vi "temp test.vi"() -> ()   [LabVIEW 2019]
doc: "This VI captures the region of the screen and displays it on the front panel continuously.\nCan be used to develop remote desktop applications."
uses:
  System.Drawing
  <vilib>/wsapi/NI_WebServices.lvlib
  <vilib>/Utility/miscctls.llb/LVBoundsTypeDef.ctl
  <vilib>/Utility/inputDevices.llb/closeMouse.vi
  <vilib>/Instr/_visa.llb/VISA Configure Serial Port (Instr).vi
  <vilib>/Utility/inputDevices.llb/mouseAcquire.vi
panel:
  out "TX":bool
  out "Scan Cycle":dbl
  out "Disable Timing":bool
  out "VISA":refnum<visa-resource-name>
  out "COM Status":bool
  in  "MC COM Port":refnum<visa-resource-name>="COM5"
  out "MLE Output":string
  out "Possible Inputs":string[](array[string])
  out "Input Likelihood":dbl[](array[numeric])
  out "Max Index":i32
  out "Write String":string
  in  "Timing Detected":bool
  out "Disable Space":bool
  out "Match Score":i32
  in  "Match Threshold":dbl=800.0
  out "Valid Range":bool
  in  "Error In 3":errorcluster
  in  "Space Detected":bool
  in  "Error In 2":errorcluster
  out "Post Processed Combo":picture
  in  "delay":u32=100
  in  "Error In":errorcluster
  out "Raw OCR Output":string
  in  "Combo y offset":i32=150
  in  "Combo x offset":i32=-100
  out "Combo":picture
  in  "Combo  Height  (px)":i32=50
  in  "Combo Width (px)":i32=360
  in  "Bar y offset":i32=200
  in  "Bar x offset":i32=-70
  out "Bar":picture
  in  "Bar Height  (px)":i32=30
  in  "Bar Width (px)":i32=280
  in  "Space Height (px)":i32=60
  in  "Space Width (px)":i32=145
  out "Space":picture
  in  "stop":bool
  # "Controls, Parameters, and Debug"
  # "Space Initiation"
  # "Bar Timing"
  # "Combo OCR"
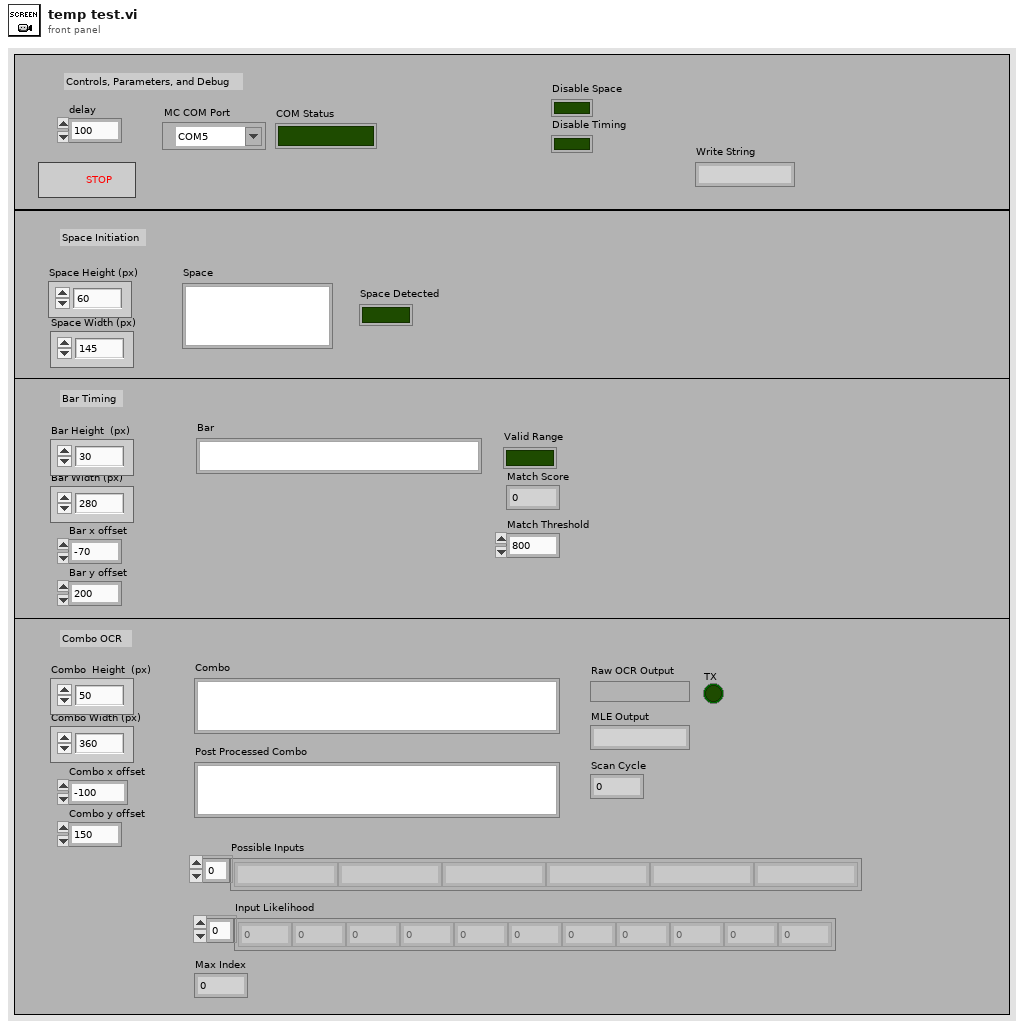
[diagram p1: front panel]
types:
  T1 = typedef "LVBoundsTypeDef.ctl" = cluster{"Width":u32, "Height":u32}
  T2 = typedef "Image Type" = u32
  T3 = cluster{"Horizontal":i32, "Vertical":i32, "Scrolling":i32}
  T4 = typedef "IMAQ Image.ctl" = refnum<image>
  T5 = typedef "imagedata.ctl" = cluster{"image type":i32, "image depth":i32, "image":u8[], "mask":u8[], "colors":u32[], "Rectangle":cluster{"left":i16, "top":i16, "right":i16, "bottom":i16}}
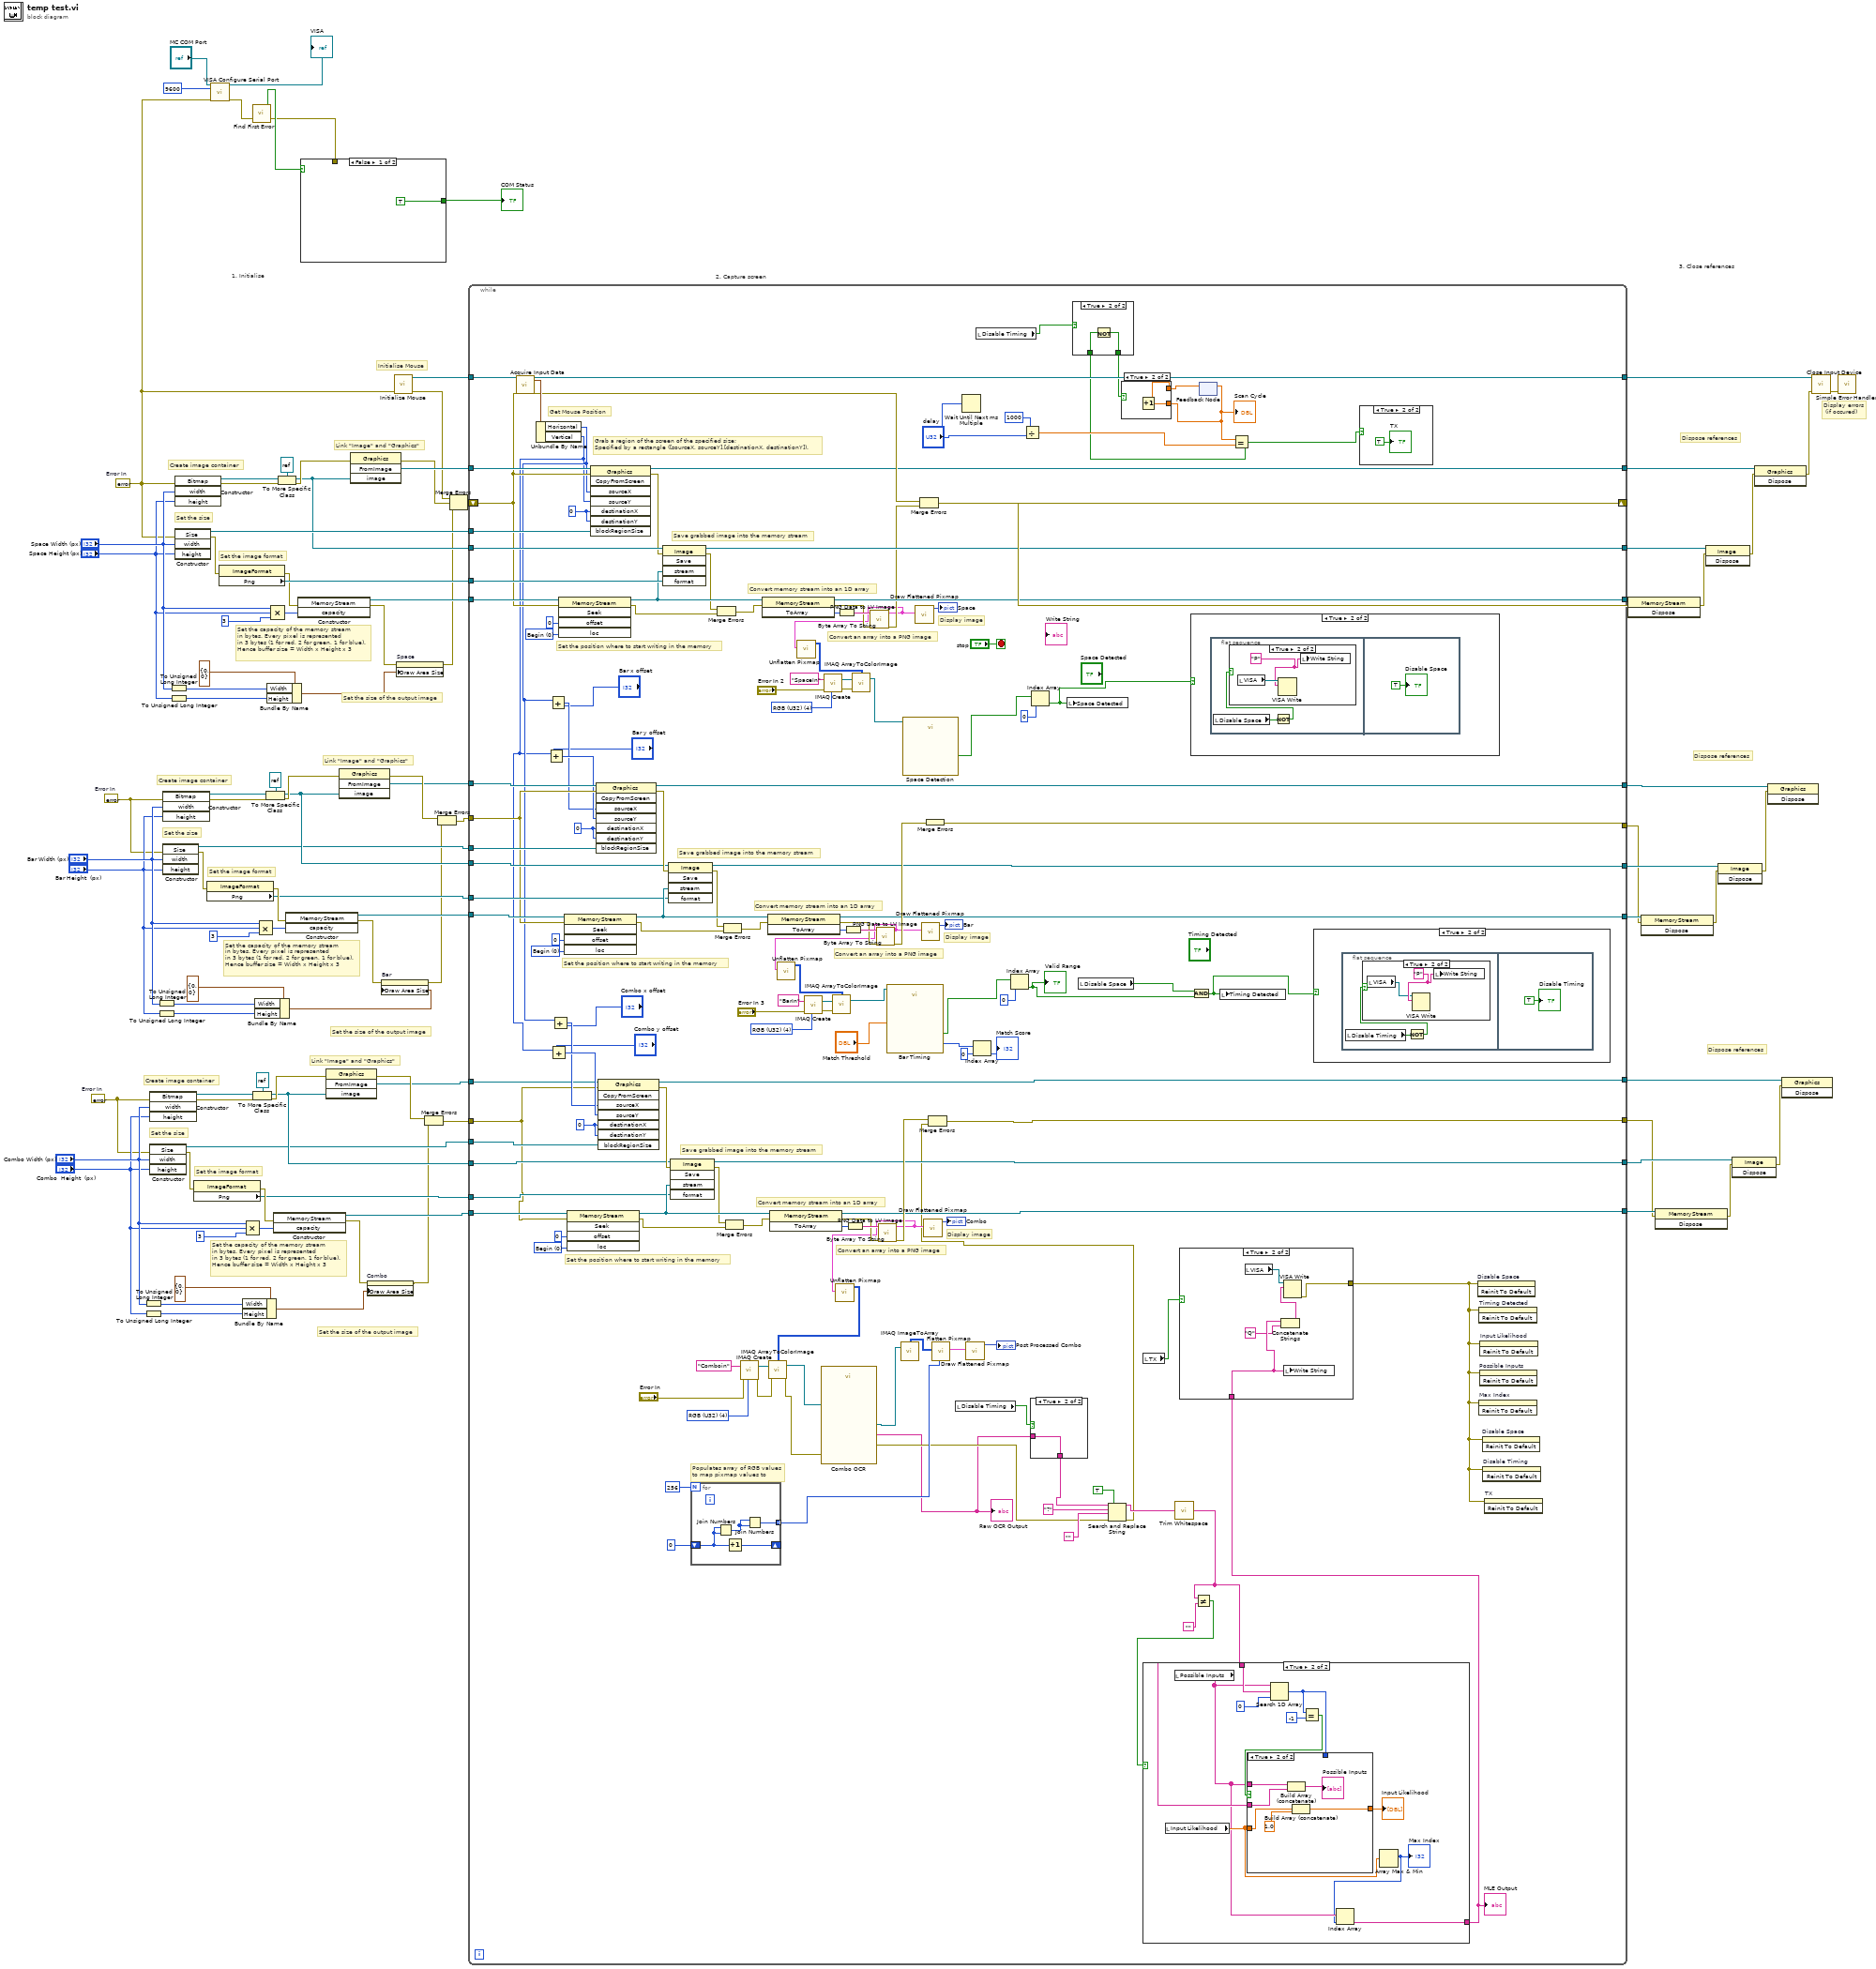
[diagram p0: block diagram]
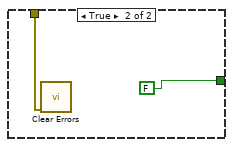
[diagram p2: hidden frame]
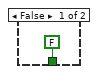
[diagram p4: hidden frame]
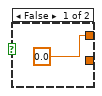
[diagram p5: hidden frame]
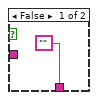
[diagram p11: hidden frame]
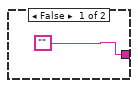
[diagram p12: hidden frame]
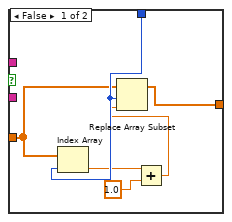
[diagram p13: hidden frame]
diagram:
  w24 = errorcluster {"status"=FALSE, "code"=0, "source"=""}  # Error In
  w54 = errorcluster {"status"=FALSE, "code"=0, "source"=""}  # Error In
  w2 = errorcluster {"status"=FALSE, "code"=0, "source"=""}  # Error In
  # "Dispose references"
  # "Link \"Image\" and \"Graphics\""
  # "Set the size"
  # "Create image container"
  # "Set the image format"
  # "Set the size of the output image"
  # "Set the capacity of the memory stream\nin bytes. Every pixel is represented\nin 3 bytes (1 for red, 2 for green, 1 for blue).\nHence buffer size = Width x Height x 3"
  # "Dispose references"
  # "Link \"Image\" and \"Graphics\""
  # "Set the size"
  # "Create image container"
  # "Set the image format"
  # "Set the size of the output image"
  # "Set the capacity of the memory stream\nin bytes. Every pixel is represented\nin 3 bytes (1 for red, 2 for green, 1 for blue).\nHence buffer size = Width x Height x 3"
  # "Link \"Image\" and \"Graphics\""
  # "Set the size"
  # "Create image container"
  # "3. Close references"
  # "2. Capture screen"
  # "1. Initialise"
  # "Display errors\n (if occured)"
  # "Dispose references"
  # "Set the image format"
  # "Set the size of the output image"
  # "Set the capacity of the memory stream\nin bytes. Every pixel is represented\nin 3 bytes (1 for red, 2 for green, 1 for blue).\nHence buffer size = Width x Height x 3"
  # "Initialise Mouse"
  n1 = To Unsigned Long Integer(number="Combo Width (px)") -> (unsigned 32bit integer=w27:u32)
  n2 = To Unsigned Long Integer(number="Combo  Height  (px)") -> (unsigned 32bit integer=w25:u32)
  n3 = constructor class="Bitmap"(error in=w24, "width"="Combo Width (px)", "height"="Combo  Height  (px)") -> (reference out=w35:refnum<k24>, error out=w37:errorcluster)  [unwired: 2 in, 3 out]
  n4 = constructor class="Size"(error in=w24, "width"="Combo Width (px)", "height"="Combo  Height  (px)") -> (reference out=w20:refnum<k24>, error out=w31:errorcluster)  [unwired: 2 in, 3 out]
  n5 = To Unsigned Long Integer(number="Bar Width (px)") -> (unsigned 32bit integer=w57:u32)
  n6 = To Unsigned Long Integer(number="Bar Height  (px)") -> (unsigned 32bit integer=w55:u32)
  n7 = constructor class="Bitmap"(error in=w54, "width"="Bar Width (px)", "height"="Bar Height  (px)") -> (reference out=w65:refnum<k24>, error out=w67:errorcluster)  [unwired: 2 in, 3 out]
  n8 = constructor class="Size"(error in=w54, "width"="Bar Width (px)", "height"="Bar Height  (px)") -> (reference out=w50:refnum<k24>, error out=w61:errorcluster)  [unwired: 2 in, 3 out]
  n9 = To Unsigned Long Integer(number="Space Width (px)") -> (unsigned 32bit integer=w76:u32)
  n10 = To Unsigned Long Integer(number="Space Height (px)") -> (unsigned 32bit integer=w74:u32)
  n11 = constructor class="Bitmap"(error in=w2, "width"="Space Width (px)", "height"="Space Height (px)") -> (reference out=w96:refnum<k24>, error out=w99:errorcluster)  [unwired: 2 in, 3 out]
  n12 = constructor class="Size"(error in=w2, "width"="Space Width (px)", "height"="Space Height (px)") -> (reference out=w94:refnum<k24>, error out=w85:errorcluster)  [unwired: 2 in, 3 out]
  n13 = property class="ImageFormat"(error in=w31) -> (error out=w30:errorcluster, "Png"=w22:refnum<k24>)  [unwired: 1 in, 1 out]
  n14 = property class="ImageFormat"(error in=w61) -> (error out=w60:errorcluster, "Png"=w52:refnum<k24>)  [unwired: 1 in, 1 out]
  n15 = call-poly "VISA Configure Serial Port"("VISA resource name"="MC COM Port", "baud rate (9600)"=u32 9600, "error in (no error)"=w2) -> ("VISA resource name out"=→"VISA":refnum<visa-resource-name>, "error out"=w7:errorcluster)  [unwired: 11 in]
  n16 = property class="ImageFormat"(error in=w85) -> (error out=w84:errorcluster, "Png"=w93:refnum<k24>)  [unwired: 1 in, 1 out]
  n17 = Bundle By Name(cluster=T1 {"Width"=0, "Height"=0} ("Draw Area Size"), "Width"=w27, "Height"=w25) -> (w11:T1)
  n18 = Compound Arithmetic op=MULTIPLY("Combo Width (px)", "Combo  Height  (px)", 3 ("value")) -> (w33:i32)
  n19 = call <vilib>:"Find First Error.vi"("error in (no error)"=w7) -> ("error out"=w4:errorcluster, "error?"=w6:bool)  [unwired: 3 in]
  n20 = To More Specific Class(target class=refnum<k24> refnum, reference=w35, error in=w37) -> (specific class reference=w21:refnum<k24>, error out=w38:errorcluster)
  n21 = Bundle By Name(cluster=T1 {"Width"=0, "Height"=0} ("Draw Area Size"), "Width"=w57, "Height"=w55) -> (w39:T1)
  n22 = Compound Arithmetic op=MULTIPLY("Bar Width (px)", "Bar Height  (px)", 3 ("value")) -> (w63:i32)
  n23 = To More Specific Class(target class=refnum<k24> refnum, reference=w65, error in=w67) -> (specific class reference=w51:refnum<k24>, error out=w68:errorcluster)
  n24 = Bundle By Name(cluster=T1 {"Width"=0, "Height"=0} ("Draw Area Size"), "Width"=w76, "Height"=w74) -> (w80:T1)
  n25 = Compound Arithmetic op=MULTIPLY("Space Width (px)", "Space Height (px)", 3 ("value")) -> (w88:i32)
  n26 = constructor class="MemoryStream"(error in=w30, "capacity"=w33) -> (reference out=w23:refnum<k24>, error out=w10:errorcluster)  [unwired: 2 in, 2 out]
  n27 = To More Specific Class(target class=refnum<k24> refnum, reference=w96, error in=w99) -> (specific class reference=w87:refnum<k24>, error out=w100:errorcluster)
  n28 = constructor class="MemoryStream"(error in=w60, "capacity"=w63) -> (reference out=w53:refnum<k24>, error out=w40:errorcluster)  [unwired: 2 in, 2 out]
  n29 = constructor class="MemoryStream"(error in=w84, "capacity"=w88) -> (reference out=w90:refnum<k24>, error out=w79:errorcluster)  [unwired: 2 in, 2 out]
  n30 = case shown="False" w6 {
    tunnel: [TRUE FALSE] -> w5
    tunnel: w4 -> [_ w104]
    frame False {
    }
    frame True {
      n31 = call <vilib>:"Clear Errors.vi"("error in (no error)"=w104) -> ()  [unwired: 5 in, 2 out]
    }
  }
  "COM Status" <- w5
  n32 = invoke class="Graphics" method="FromImage"(error in=w38, "image"=w21) -> (error out=w29:errorcluster, "FromImage"=w19:refnum<k24>)  [unwired: 2 in, 2 out]
  n33 = invoke class="Graphics" method="FromImage"(error in=w68, "image"=w51) -> (error out=w59:errorcluster, "FromImage"=w49:refnum<k24>)  [unwired: 2 in, 2 out]
  n34 = invoke class="Graphics" method="FromImage"(error in=w100, "image"=w87) -> (error out=w83:errorcluster, "FromImage"=w97:refnum<k24>)  [unwired: 2 in, 2 out]
  n35 = property on="Combo" class="Pict"(error in=w10, "Draw Area Size"=w11) -> (error out=w9:errorcluster)  [unwired: 1 in, 1 out]
  n36 = property on="Bar" class="Pict"(error in=w40, "Draw Area Size"=w39) -> (error out=w41:errorcluster)  [unwired: 1 in, 1 out]
  n37 = call <vilib>:"Initialize Mouse.vi"("error in (no error)"=w2) -> ("error out"=w81:errorcluster, "device ID"=w102:refnum<k1>)  [unwired: 9 in]
  n38 = property on="Space" class="Pict"(error in=w79, "Draw Area Size"=w80) -> (error out=w78:errorcluster)  [unwired: 1 in, 1 out]
  n39 = Merge Errors(w29, w9) -> (w18:errorcluster)
  n40 = Merge Errors(w59, w41) -> (w48:errorcluster)
  n41 = Merge Errors(w81, w83, w78) -> (w82:errorcluster)
  n42 = while {
    tunnel: w102 -> [w256]
    tunnel: [w254] -> w101
    tunnel: w97 -> [w253]
    tunnel: [w250] -> w95
    tunnel: w94 -> [w249]
    tunnel: w93 -> [w248]
    tunnel: [w247] -> w92
    tunnel: w90 -> [w246]
    tunnel: w87 -> [w239]
    shift-right: [w230] -> w73
    shift-left: w82 -> [w233]
    tunnel: [w229] -> w72
    tunnel: w53 -> [w215]
    tunnel: w52 -> [w214]
    tunnel: w51 -> [w213]
    tunnel: w50 -> [w212]
    tunnel: w49 -> [w211]
    tunnel: w48 -> [w210]
    tunnel: [w209] -> w45
    tunnel: [w208] -> w44
    tunnel: [w207] -> w43
    tunnel: [w206] -> w42
    tunnel: w23 -> [w184]
    tunnel: w22 -> [w183]
    tunnel: w21 -> [w182]
    tunnel: w20 -> [w181]
    tunnel: w19 -> [w180]
    tunnel: w18 -> [w179]
    tunnel: [w176] -> w15
    tunnel: [w175] -> w14
    tunnel: [w174] -> w13
    tunnel: [w173] -> w12
    stop <- "stop" stop-if-true
    w146 = T2 4 items=["Grayscale (U8)", "Grayscale (I16)", "Grayscale (SGL)", "Complex (CSG)", "RGB (U32)", "HSL (U32)", "RGB (U64)", "Grayscale (U16)"] ("Image Type")
    w157 = T2 4 items=["Grayscale (U8)", "Grayscale (I16)", "Grayscale (SGL)", "Complex (CSG)", "RGB (U32)", "HSL (U32)", "RGB (U64)", "Grayscale (U16)"] ("Image Type")
    w172 = T2 4 items=["Grayscale (U8)", "Grayscale (I16)", "Grayscale (SGL)", "Complex (CSG)", "RGB (U32)", "HSL (U32)", "RGB (U64)", "Grayscale (U16)"] ("Image Type")
    w195 = 0 ("destinationX")
    w198 = 0 items=["Begin", "Current", "End"] ("loc")
    w222 = 0 ("destinationX")
    w225 = 0 items=["Begin", "Current", "End"] ("loc")
    w240 = 0 ("destinationX")
    w244 = 0 items=["Begin", "Current", "End"] ("loc")
    # "Populates array of RGB values\nto map pixmap values to"
    # "Display image"
    # "Convert an array into a PNG image"
    # "Set the position where to start writing in the memory"
    # "Convert memory stream into an 1D array"
    # "Save grabbed image into the memory stream"
    # "Display image"
    # "Convert an array into a PNG image"
    # "Set the position where to start writing in the memory"
    # "Convert memory stream into an 1D array"
    # "Save grabbed image into the memory stream"
    # "Display image"
    # "Convert an array into a PNG image"
    # "Set the position where to start writing in the memory"
    # "Convert memory stream into an 1D array"
    # "Save grabbed image into the memory stream"
    # "Grab a region of the screen of the specified size;\nSpecified by a rectangle ([sourceX, sourceY],[destinationX, destinationY])."
    # "Get Mouse Position"
    n43 = call-poly <vilib>:"Acquire Input Data.vi"("device ID"=w256, "error in (no error)"=w233) -> ("device ID"=w254:refnum<k1>, "axis info"=w255:T3, "error out"=w232:errorcluster)  [unwired: 14 in, 1 out]
    n44 = Unbundle By Name(w255) -> ("Horizontal"=w178:i32, "Vertical"=w177:i32)
    n45 = Add(x=w177, y="Bar y offset") -> (x+y=w205:i32)
    n46 = Add(x=w178, y="Bar x offset") -> (x+y=w204:i32)
    n47 = Add(x=w177, y="Combo y offset") -> (x+y=w188:i32)
    n48 = Add(x=w178, y="Combo x offset") -> (x+y=w187:i32)
    n49 = invoke class="MemoryStream" method="Seek"(reference=w246, error in=w233, "offset"=i64 0, "loc"=w244) -> (reference out=w241:refnum<k24>, error out=w236:errorcluster)  [unwired: 1 in, 3 out]
    n50 = invoke class="MemoryStream" method="Seek"(reference=w215, error in=w210, "offset"=i64 0, "loc"=w225) -> (reference out=w223:refnum<k24>, error out=w219:errorcluster)  [unwired: 1 in, 3 out]
    n51 = invoke class="MemoryStream" method="Seek"(reference=w184, error in=w179, "offset"=i64 0, "loc"=w198) -> (reference out=w196:refnum<k24>, error out=w192:errorcluster)  [unwired: 1 in, 3 out]
    n52 = invoke class="Graphics" method="CopyFromScreen"(reference=w253, error in=w233, "sourceX"=w178, "sourceY"=w177, "destinationX"=w240, "destinationY"=w240, "blockRegionSize"=w249) -> (reference out=w229:refnum<k24>, error out=w234:errorcluster)  [unwired: 1 in, 6 out]
    n53 = invoke class="Graphics" method="CopyFromScreen"(reference=w211, error in=w210, "sourceX"=w204, "sourceY"=w205, "destinationX"=w222, "destinationY"=w222, "blockRegionSize"=w212) -> (reference out=w208:refnum<k24>, error out=w217:errorcluster)  [unwired: 1 in, 6 out]
    n54 = invoke class="Graphics" method="CopyFromScreen"(reference=w180, error in=w179, "sourceX"=w187, "sourceY"=w188, "destinationX"=w195, "destinationY"=w195, "blockRegionSize"=w181) -> (reference out=w173:refnum<k24>, error out=w190:errorcluster)  [unwired: 1 in, 6 out]
    n55 = invoke class="Image" method="Save"(reference=w239, error in=w234, "stream"=w241, "format"=w248) -> (reference out=w247:refnum<k24>, error out=w237:errorcluster)  [unwired: 1 in, 3 out]
    n56 = invoke class="Image" method="Save"(reference=w213, error in=w217, "stream"=w223, "format"=w214) -> (reference out=w209:refnum<k24>, error out=w220:errorcluster)  [unwired: 1 in, 3 out]
    n57 = invoke class="Image" method="Save"(reference=w182, error in=w190, "stream"=w196, "format"=w183) -> (reference out=w175:refnum<k24>, error out=w193:errorcluster)  [unwired: 1 in, 3 out]
    n58 = for {
      N: 256 -> [_]
      tunnel: [w307] -> w158 mode=indexing
      shift-right: [w306] -> _
      shift-left: u8 0 -> [w304]
      n59 = Join Numbers(hi=w304, lo=w304) -> ((hi.lo)=w305:u16)
      n60 = Increment(x=w304) -> (x+1=w306:u8)
      n61 = Join Numbers(hi=w305, lo=w305) -> ((hi.lo)=w307:u32)
    }
    n62 = Merge Errors(w237, w236) -> (w235:errorcluster)
    n63 = Merge Errors(w220, w219) -> (w218:errorcluster)
    n64 = Merge Errors(w193, w192) -> (w191:errorcluster)
    n65 = call "IMAQ Create"("Image Name"="Comboin", "Image Type"=w172, "error in (no error)"="Error In") -> ("New Image"=w171:T4, "error out"=w170:errorcluster)  [unwired: 1 in, 1 out]
    n66 = invoke class="MemoryStream" method="ToArray"(reference=w241, error in=w235) -> (reference out=w250:refnum<k24>, error out=w238:errorcluster, "ToArray"=w252:u8[])  [unwired: 1 in]
    n67 = invoke class="MemoryStream" method="ToArray"(reference=w223, error in=w218) -> (reference out=w207:refnum<k24>, error out=w221:errorcluster, "ToArray"=w228:u8[])  [unwired: 1 in]
    n68 = invoke class="MemoryStream" method="ToArray"(reference=w196, error in=w191) -> (reference out=w176:refnum<k24>, error out=w194:errorcluster, "ToArray"=w201:u8[])  [unwired: 1 in]
    n69 = call "IMAQ Create"("Image Name"="BarIn", "Image Type"=w146, "error in (no error)"="Error In 3") -> ("New Image"=w145:T4, "error out"=w144:errorcluster)  [unwired: 1 in, 1 out]
    n70 = call "IMAQ Create"("Image Name"="SpaceIn", "Image Type"=w157, "error in (no error)"="Error In 2") -> ("New Image"=w156:T4, "error out"=w155:errorcluster)  [unwired: 1 in, 1 out]
    n71 = Byte Array To String(unsigned byte array=w252) -> (string=w251:string)
    n72 = Byte Array To String(unsigned byte array=w228) -> (string=w227:string)
    n73 = Byte Array To String(unsigned byte array=w201) -> (string=w200:string)
    n74 = call <vilib>:"PNG Data to LV Image.vi"("error in (no error)"=w238, "png data"=w251) -> ("error out"=w231:errorcluster, "image data"=w153:T5)  [unwired: 8 in]
    n75 = call <vilib>:"Unflatten Pixmap.vi"("image data"=w153) -> ("24-bit pixmap"=w152:u32[][])  [unwired: 4 in, 6 out]
    n76 = call "IMAQ ArrayToColorImage"("Image Pixels (U32)"=w152, "Image"=w156, "error in (no error)"=w155) -> ("Image Out"=w151:T4)  [unwired: 2 in, 1 out]
    n77 = call <vilib>:"PNG Data to LV Image.vi"("error in (no error)"=w221, "png data"=w227) -> ("error out"=w216:errorcluster, "image data"=w140:T5)  [unwired: 8 in]
    n78 = call <vilib>:"Unflatten Pixmap.vi"("image data"=w140) -> ("24-bit pixmap"=w139:u32[][])  [unwired: 4 in, 6 out]
    n79 = call "IMAQ ArrayToColorImage"("Image Pixels (U32)"=w139, "Image"=w145, "error in (no error)"=w144) -> ("Image Out"=w141:T4)  [unwired: 2 in, 1 out]
    n80 = call <vilib>:"PNG Data to LV Image.vi"("error in (no error)"=w194, "png data"=w200) -> ("error out"=w189:errorcluster, "image data"=w167:T5)  [unwired: 8 in]
    n81 = call <vilib>:"Unflatten Pixmap.vi"("image data"=w167) -> ("24-bit pixmap"=w166:u32[][])  [unwired: 4 in, 6 out]
    n82 = call "IMAQ ArrayToColorImage"("Image Pixels (U32)"=w166, "Image"=w171, "error in (no error)"=w170) -> ("Image Out"=w168:T4, "error out"=w169:errorcluster)  [unwired: 2 in]
    n83 = call "Combo OCR"("Image In"=w168, "error in"=w169) -> ("Image Out"=w164:T4, "String (OCR/OCV 2)"=w120:string, "error out"=w128:errorcluster)  [unwired: 23 in]
    "Raw OCR Output" <- w120
    n84 = call "Bar Timing"("Image In"=w141, "Minimum Match Score (Color Matching 1)"="Match Threshold") -> ("Match Flag (Color Matching 1)"=w137:bool[], "Match Score (Color Matching 1)"=w135:i32[])  [unwired: 22 in, 2 out]
    n85 = call "IMAQ ImageToArray"("Image"=w164) -> ("Image Pixels (U8)"=w161:u8[][])  [unwired: 3 in, 4 out]
    n86 = call "Space Detection"("Image In"=w151) -> ("Match Flag (Color Matching 1)"=w148:bool[])  [unwired: 23 in, 3 out]
    n87 = call <vilib>:"Draw Flattened Pixmap.vi"("image data"=w153) -> ("new picture"=→"Space":picture)  [unwired: 8 in]
    n88 = Merge Errors(w232, w231) -> (w230:errorcluster)
    n89 = call <vilib>:"Draw Flattened Pixmap.vi"("image data"=w140) -> ("new picture"=→"Bar":picture)  [unwired: 8 in]
    n90 = call <vilib>:"Draw Flattened Pixmap.vi"("image data"=w167) -> ("new picture"=→"Combo":picture)  [unwired: 8 in]
    n91 = Merge Errors(w216) -> (w206:errorcluster)
    n92 = call <vilib>:"Flatten Pixmap.vi"("colors"=w158, "8-bit pixmap"=w161) -> ("image data"=w162:T5)  [unwired: 9 in]
    n93 = local read "Disable Timing"() -> (w109:bool)
    n94 = Wait Until Next ms Multiple(millisecond multiple="delay") -> ()  [unwired: 1 out]
    n95 = call <vilib>:"Draw Flattened Pixmap.vi"("image data"=w162) -> ("new picture"=→"Post Processed Combo":picture)  [unwired: 8 in]
    n96 = Index Array(array=w135, index=0) -> (element=→"Match Score":i32)
    n97 = local read "Disable Timing"() -> (w110:bool)
    n98 = Index Array(array=w137, index=0) -> (element=w123:bool)
    "Valid Range" <- w123
    n99 = Divide(x=1000, y="delay") -> (x/y=w116:dbl)
    n100 = case shown="True" w109 {
      tunnel: ["" w280] -> w121
      tunnel: w120 -> [_ w280]
      frame False {
      }
      frame True {
      }
    }
    n101 = Index Array(array=w148, index=0) -> (element=w117:bool)
    n102 = local write "Space Detected"(w117) -> ()
    n103 = local read "Disable Space"() -> (w122:bool)
    n104 = Search and Replace String(replace all?=TRUE ("replace all? (F)"), input string=w121, search string="?", replace string="", error in=w128) -> (result string=w129:string, error out=w127:errorcluster)  [unwired: 3 in, 2 out]
    n105 = Merge Errors(w189, w127) -> (w174:errorcluster)
    n106 = local read "TX"() -> (w107:bool)
    n107 = call <vilib>:"Trim Whitespace.vi"("string"=w129) -> ("trimmed string"=w125:string)  [unwired: 1 in]
    n108 = case shown="True" w117 {
      frame False {
      }
      frame True {
        n109 = flat-sequence {
          frame #0 {
            n110 = local read "Disable Space"() -> (w265:bool)
            n111 = Not(x=w265) -> (.not. x?=w264:bool)
            n112 = case shown="True" w264 {
              frame False {
              }
              frame True {
                w266 = "P" ("Write String")
                n113 = local read "VISA"() -> (w267:refnum<visa-resource-name>)
                n114 = VISA Write(VISA resource name=w267, write buffer=w266) -> ()  [unwired: 1 in, 3 out]
                n115 = local write "Write String"(w266) -> ()
              }
            }
          }
          frame #1 {
            "Disable Space" <- TRUE ("Enable Space")
          }
        }
      }
    }
    n116 = And(x=w122, y=w123) -> (x .and. y?=w118:bool)
    n117 = Not Equal?(x=w125, y="") -> (x != y?=w124:bool)
    n118 = case shown="True" w124 {
      tunnel: w125 -> [_ w286]
      tunnel: ["" w282] -> w119
      frame False {
      }
      frame True {
        n119 = local read "Input Likelihood"() -> (w285:dbl[])
        n120 = local read "Possible Inputs"() -> (w284:string[])
        n121 = Search 1D Array(1D array=w284, element=w286, start index (0)=0) -> (index of element=w288:i32)
        n122 = Equal?(x=w288, y=-1) -> (x = y?=w289:bool)
        n123 = case shown="True" w289 {
          tunnel: w284 -> [_ w303]
          tunnel: w286 -> [_ w302]
          tunnel: w288 -> [w297 _]
          tunnel: w285 -> [w293 w299]
          tunnel: [w292 w300] -> w287
          frame False {
            n124 = Index Array(array=w293, index=w297) -> (element=w295:dbl)
            n125 = Add(x=w295, y=1.0) -> (x+y=w294:dbl)
            n126 = Replace Array Subset(array=w293, new element=w294, index=w297) -> (w292:dbl[])
          }
          frame True {
            n127 = Build Array (concatenate)(w303, w302) -> (→"Possible Inputs":string[])
            n128 = Build Array (concatenate)(w299, 1.0 ("new element/subarray")) -> (w300:dbl[])
          }
        }
        "Input Likelihood" <- w287
        n129 = Array Max & Min(array=w285) -> (max index (indices)=w283:i32)  [unwired: 3 out]
        "Max Index" <- w283
        n130 = Index Array(array=w284, index=w283) -> (element=w282:string)
      }
    }
    "MLE Output" <- w119
    n131 = case shown="True" w107 {
      tunnel: w119 -> [_ w273]
      tunnel: [_ w269] -> w106
      frame False {
      }
      frame True {
        n132 = local read "VISA"() -> (w272:refnum<visa-resource-name>)
        n133 = Concatenate Strings(w273, "Q" ("string")) -> (w270:string)
        n134 = VISA Write(VISA resource name=w272, write buffer=w270) -> (error out=w269:errorcluster)  [unwired: 1 in, 2 out]
        n135 = local write "Write String"(w273) -> ()
      }
    }
    n136 = feedback #1() -> (w115:dbl)  [unwired: 1 in]
    "Scan Cycle" <- w115
    n137 = local write "Timing Detected"(w118) -> ()
    n138 = Equal?(x=w115, y=w116) -> (x = y?=w108:bool)
    n139 = case shown="True" w110 {
      tunnel: [FALSE w260] -> w114
      tunnel: w108 -> [_ w259]
      frame False {
      }
      frame True {
        n140 = Not(x=w259) -> (.not. x?=w260:bool)
      }
    }
    n141 = case shown="True" w114 {
      tunnel: [0.0 w263] -> w112
      tunnel: w115 -> [_ w262]
      frame False {
      }
      frame True {
        n142 = Increment(x=w262) -> (x+1=w263:dbl)
      }
    }
    n143 = feedback-in #1(w112) -> ()
    n144 = case shown="True" w118 {
      frame False {
      }
      frame True {
        n145 = flat-sequence {
          frame #0 {
            n146 = local read "Disable Timing"() -> (w275:bool)
            n147 = Not(x=w275) -> (.not. x?=w274:bool)
            n148 = case shown="True" w274 {
              frame False {
              }
              frame True {
                w277 = "P" ("Write String")
                n149 = local read "VISA"() -> (w276:refnum<visa-resource-name>)
                n150 = VISA Write(VISA resource name=w276, write buffer=w277) -> ()  [unwired: 1 in, 3 out]
                n151 = local write "Write String"(w277) -> ()
              }
            }
          }
          frame #1 {
            "Disable Timing" <- TRUE ("Enable Space")
          }
        }
      }
    }
    n152 = case shown="True" w108 {
      frame False {
      }
      frame True {
        "TX" <- TRUE ("TX")
      }
    }
    n153 = invoke on="Disable Space" class="Bool (strict)" method="Reinit To Default"(error in=w106) -> ()  [unwired: 2 in, 3 out]
    n154 = invoke on="Timing Detected" class="Bool (strict)" method="Reinit To Default"(error in=w106) -> ()  [unwired: 2 in, 3 out]
    n155 = invoke on="Max Index" class="DigNum (strict)" method="Reinit To Default"(error in=w106) -> ()  [unwired: 2 in, 3 out]
    n156 = invoke on="Possible Inputs" class="Arr (strict)" method="Reinit To Default"(error in=w106) -> ()  [unwired: 2 in, 3 out]
    n157 = invoke on="Input Likelihood" class="Arr (strict)" method="Reinit To Default"(error in=w106) -> ()  [unwired: 2 in, 3 out]
    n158 = invoke on="Disable Space" class="Bool (strict)" method="Reinit To Default"(error in=w106) -> ()  [unwired: 2 in, 3 out]
    n159 = invoke on="Disable Timing" class="Bool (strict)" method="Reinit To Default"(error in=w106) -> ()  [unwired: 2 in, 3 out]
    n160 = invoke on="TX" class="Bool (strict)" method="Reinit To Default"(error in=w106) -> ()  [unwired: 2 in, 3 out]
  }
  n161 = invoke class="MemoryStream" method="Dispose"(reference=w95, error in=w73) -> (error out=w91:errorcluster)  [unwired: 1 in, 2 out]
  n162 = invoke class="MemoryStream" method="Dispose"(reference=w43, error in=w42) -> (error out=w47:errorcluster)  [unwired: 1 in, 2 out]
  n163 = invoke class="MemoryStream" method="Dispose"(reference=w15, error in=w13) -> (error out=w17:errorcluster)  [unwired: 1 in, 2 out]
  n164 = invoke class="Image" method="Dispose"(reference=w92, error in=w91) -> (error out=w71:errorcluster)  [unwired: 1 in, 2 out]
  n165 = invoke class="Image" method="Dispose"(reference=w45, error in=w47) -> (error out=w46:errorcluster)  [unwired: 1 in, 2 out]
  n166 = invoke class="Image" method="Dispose"(reference=w14, error in=w17) -> (error out=w16:errorcluster)  [unwired: 1 in, 2 out]
  n167 = invoke class="Graphics" method="Dispose"(reference=w72, error in=w71) -> (error out=w70:errorcluster)  [unwired: 1 in, 2 out]
  n168 = invoke class="Graphics" method="Dispose"(reference=w44, error in=w46) -> ()  [unwired: 1 in, 3 out]
  n169 = invoke class="Graphics" method="Dispose"(reference=w12, error in=w16) -> ()  [unwired: 1 in, 3 out]
  n170 = call-poly <vilib>:"Close Input Device.vi"("error in (no error)"=w70, "device ID"=w101) -> ("error out"=w69:errorcluster)  [unwired: 8 in]
  n171 = call <vilib>:"Simple Error Handler.vi"("error in (no error)"=w69) -> ()  [unwired: 4 in, 5 out]
